vi "programa7.vi"() -> ()   [LabVIEW 2011]
panel:
  out "Contador":dbl
  out "Mayores a 50":dbl
  out "Suma":dbl
  out "Numero":dbl
  # "Ciclo While"
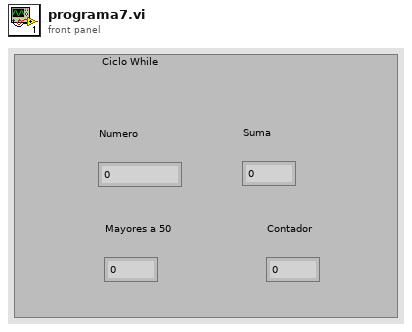
[diagram p1: front panel]
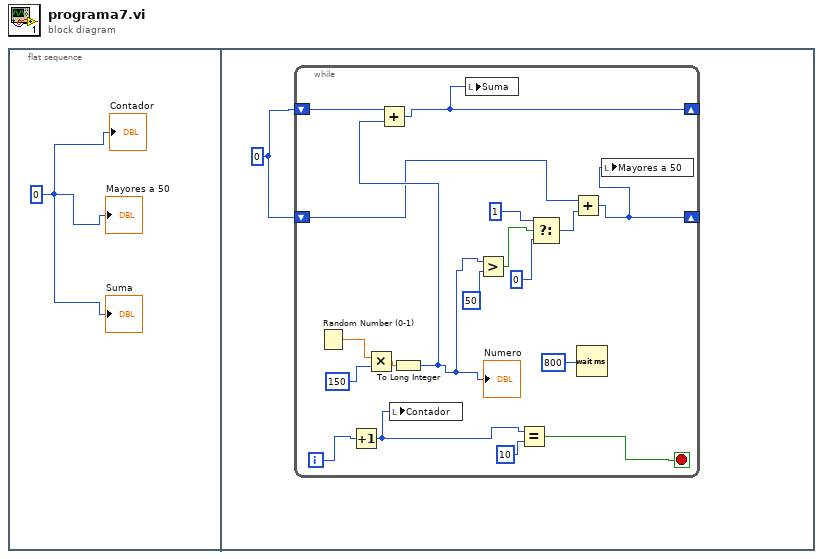
[diagram p0: block diagram]
diagram:
  n1 = flat-sequence {
    frame #0 {
      w1 = 0
      "Suma" <- w1
      "Mayores a 50" <- w1
      "Contador" <- w1
    }
    frame #1 {
      w2 = 0
      n2 = while {
        shift-right: [w11] -> _
        shift-left: w2 -> [w12]
        shift-right: [w3] -> _
        shift-left: w2 -> [w4]
        i -> [w20]
        stop <- w18 stop-if-true
        n3 = Random Number (0-1)() -> (number: 0 to 1=w16:dbl)
        n4 = Increment(x=w20) -> (x+1=w13:i32)
        n5 = Multiply(x=w16, y=150) -> (x*y=w15:dbl)
        n6 = local write "Contador"(w13) -> ()
        n7 = To Long Integer(number=w15) -> (32bit integer=w10:i32)
        "Numero" <- w10
        n8 = Add(x=w12, y=w10) -> (x+y=w11:i32)
        n9 = local write "Suma"(w11) -> ()
        n10 = Greater?(x=w10, y=50) -> (0:w8:bool)
        n11 = Equal?(x=w13, y=10) -> (x = y?=w18:bool)
        n12 = Select(t=1, s=w8, f=0) -> (s? t:f=w5:i32)
        n13 = Add(x=w4, y=w5) -> (x+y=w3:i32)
        n14 = Wait (ms)(milliseconds to wait=800) -> ()  [unwired: 1 out]
        n15 = local write "Mayores a 50"(w3) -> ()
      }
    }
  }
